vi "Read Dev.TCPIP.EthernetMAC.vi"(8 "error in (no error)":errorcluster, 11 "SLSC Interface in":refnum<class "SLSC Interface.lvclass">) -> (0 "error out":errorcluster, 2 "Dev.TCPIP.EthernetMAC":string, 3 "SLSC Interface out":refnum<class "SLSC Interface.lvclass">)   [LabVIEW 2015, in "SLSC Interface.lvclass"]
uses:
  SLSC Interface.lvclass
  SLSC Interface.lvclass/SLSC Interface.ctl
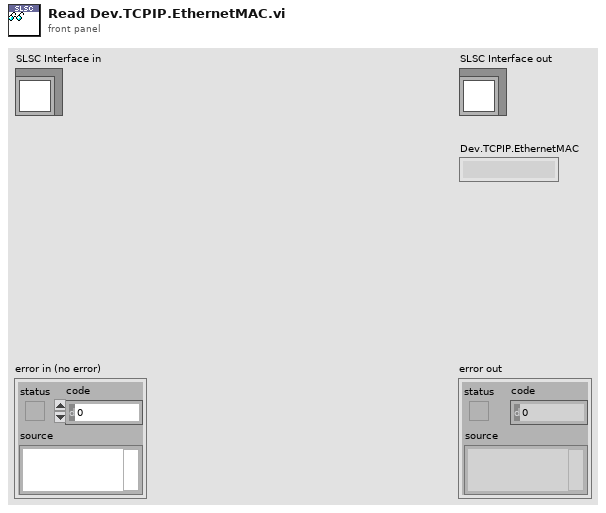
[diagram p1: front panel]
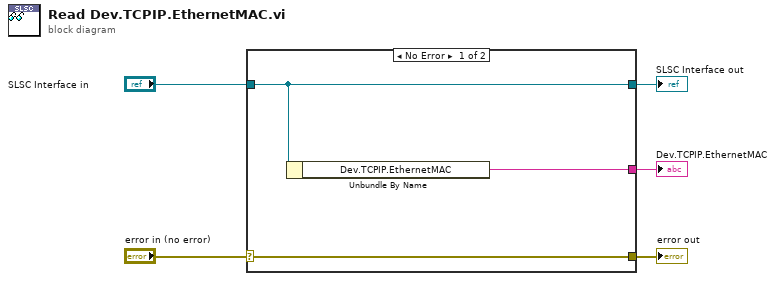
[diagram p0: block diagram]
diagram:
  n1 = case shown="No Error" "error in (no error)" {
    selector: "error in (no error)" -> [w8 w9]
    tunnel: [w8 w9] -> w4
    tunnel: [w7 w10] -> w2
    tunnel: "SLSC Interface in" -> [w7 w10]
    tunnel: [w6 _] -> w1
    frame No Error {
      n2 = Unbundle By Name(w7) -> ("Dev.TCPIP.EthernetMAC"=w6:string)
    }
    frame Error {
    }
  }
  "error out" <- w4
  "SLSC Interface out" <- w2
  "Dev.TCPIP.EthernetMAC" <- w1
